vi "Update_PKYK.vi"(8 "error in (no error)":errorcluster, 10 "PokaYoke In":T1 {"MachineCode" items=["MCIG", "MCPC", "MCSA", "MCCA", "MCAC", "MCLA", "MCCM", "MCSC", "MCPA", "MCLP", "MCHP", "MCBC", "MCFA", "MCSR", "MCFV"]; "ExpiryDate" format="%<%I:%M:%S%3u %p\n%d-%m-%Y>T"; "EntDt" format="%<%I:%M:%S%3u %p\n%d-%m-%Y>T"; "UpdDt" format="%<%I:%M:%S%3u %p\n%d-%m-%Y>T"}, 11 "Refnum in":T6) -> (0 "error out":errorcluster, 2 "PokaYoke Out":T1 {"MachineCode" items=["MCIG", "MCPC", "MCSA", "MCCA", "MCAC", "MCLA", "MCCM", "MCSC", "MCPA", "MCLP", "MCHP", "MCBC", "MCFA", "MCSR", "MCFV"]; "ExpiryDate" format="%<%I:%M:%S%3u %p\n%d-%m-%Y>T"; "EntDt" format="%<%I:%M:%S%3u %p\n%d-%m-%Y>T"; "UpdDt" format="%<%I:%M:%S%3u %p\n%d-%m-%Y>T"}, 3 "Refnum out":T6)   [LabVIEW 2020]
uses:
  <vilib>/addons/database/Connection.llb/Conn ObjectReference.ctl
  Controls/Line_PKYK.ctl
  Controls/PARA_CONTROL_STR.ctl
  Controls/PKYK_MCODE.ctl
  Controls/PKYK_DATE.ctl
  Controls/PKYK_Result.ctl
  <userlib>/_OpenG.lib/array/array.llb/Delete Elements from 1D Array (String)__ogtk.vi
  <vilib>/addons/database/NI_Database_API.lvlib
panel:
  out "Format String Name":string[](array[string])
  out "resulting string":string
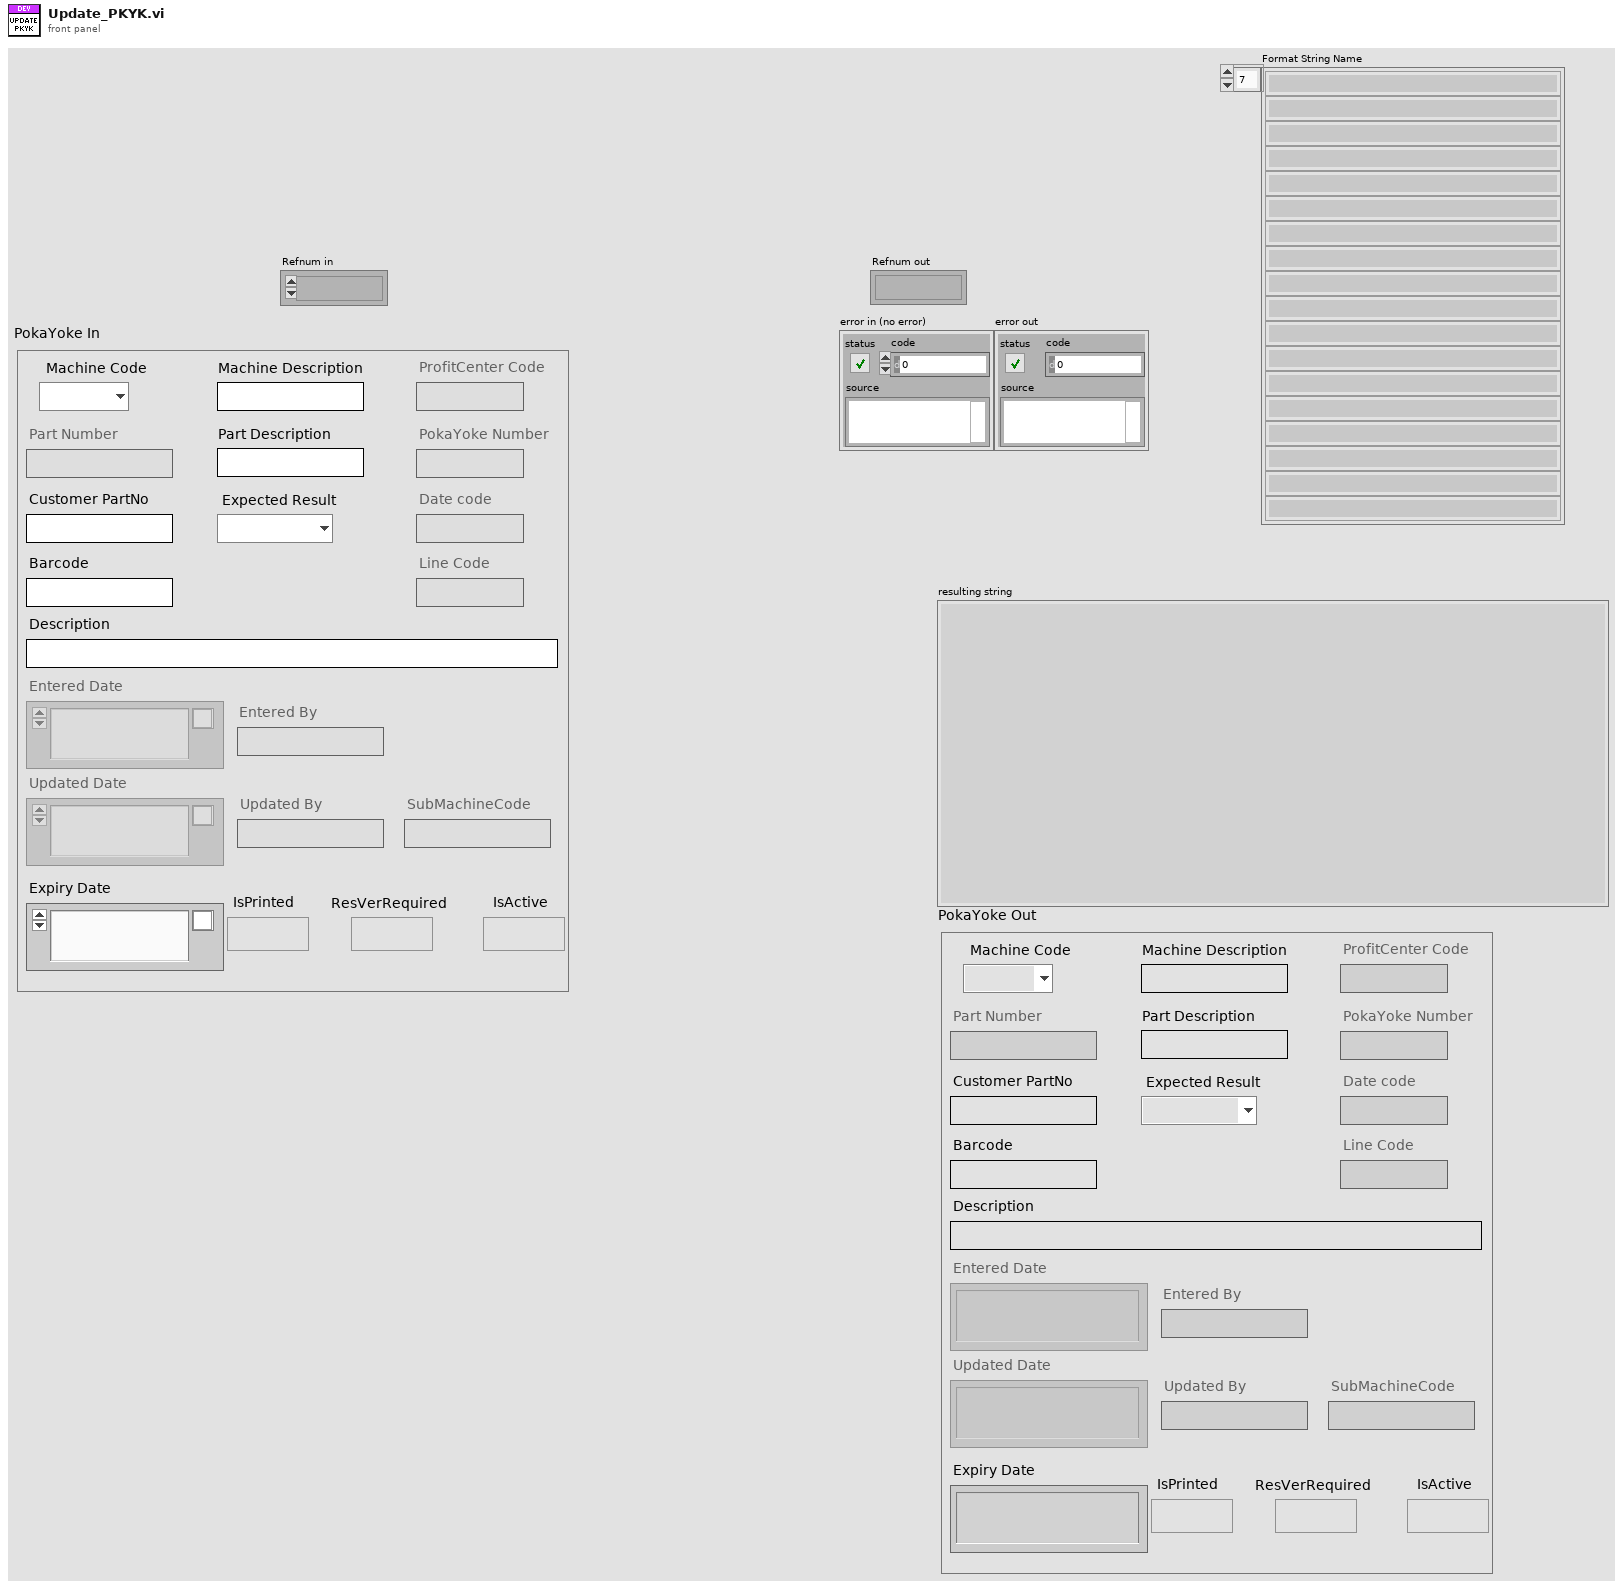
[diagram p1: front panel]
types:
  T1 = typedef "Line_PKYK.ctl" = cluster{"ProfitCenterCode":string, "LineCode":string, "Datecode":string, "PartNumber":T2, "PartDescription":T2, "CustPartNo":T2, "MachineCode":T3, "MachineDescription":T2, "PokaYokeNumber":string, "Description":string, "ExpiryDate":T4, "Barcode":T2, "IsPrinted":bool, "IsActive":bool, "EntBy":T2, "EntDt":T4, "UpdBy":T2, "UpdDt":T4, "ExpResult":T5, "ResVerRequired":bool, "SubMachineCode":T2}
  T2 = typedef "PARA_CONTROL_STR.ctl" = string
  T3 = typedef "PKYK_MCODE.ctl" = u16
  T4 = typedef "PKYK_DATE.ctl" = timestamp
  T5 = typedef "PKYK_Result.ctl" = enum16{"FAIL", "PASS"}
  T6 = typedef "NI_Database_API.lvlib/Conn ObjectReference.ctl" = refnum<k1>
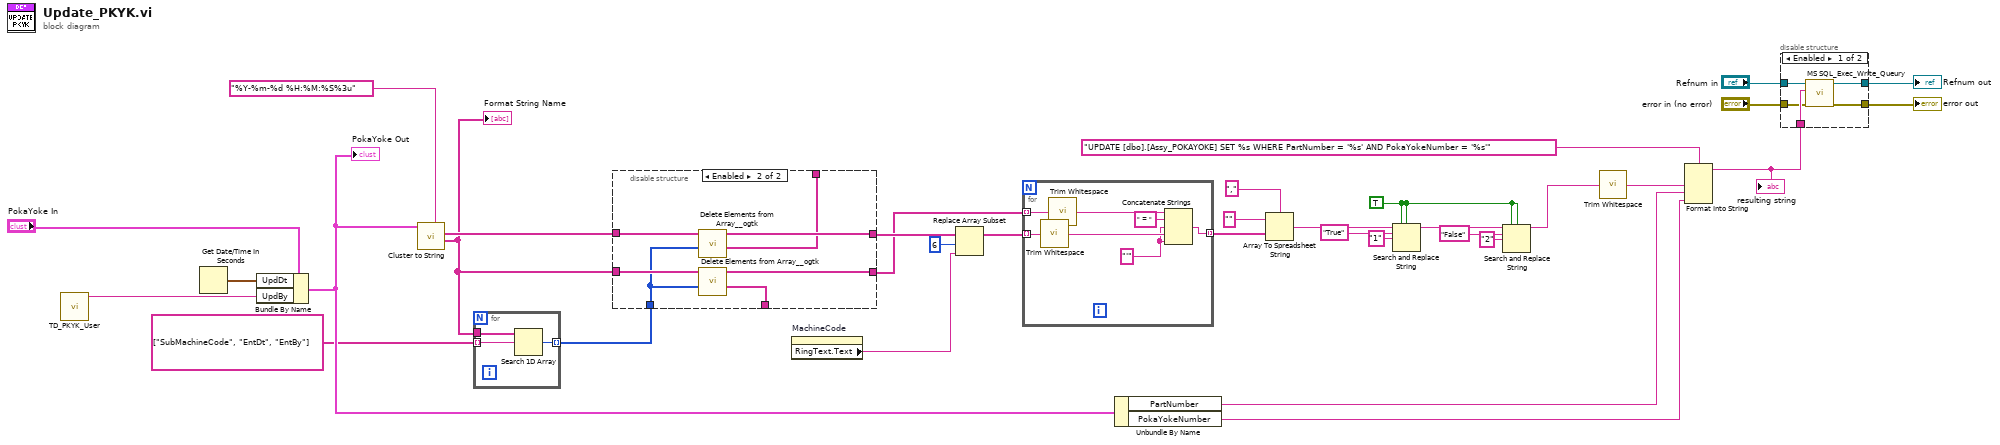
[diagram p0: block diagram]
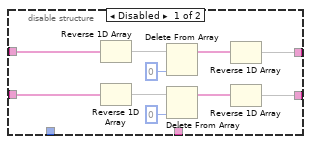
[diagram p2: hidden frame]
diagram:
  w28 = TRUE ("replace all? (F)")
  n1 = call "TD_PKYK_User.vi"() -> ("User"=w1:string)  [unwired: 11 in]
  n2 = Get Date/Time In Seconds() -> (seconds since 1Jan1904=w11:timestamp)
  n3 = Bundle By Name(cluster="PokaYoke In", "UpdDt"=w11, "UpdBy"=w1) -> (w7:T1)
  "PokaYoke Out" <- w7
  n4 = call <userlib>:"Cluster to String.vi"("Time Format String"="%Y-%m-%d %H:%M:%S%3u" ("time format string (%c)"), "Variant In"=w7) -> ("Format String Name"=w4:string[], "Format String Array"=w13:string[])  [unwired: 6 in, 2 out]
  "Format String Name" <- w4
  n5 = for {
    tunnel: w4 -> [w37]
    tunnel: string[] ["SubMachineCode", "EntDt", "EntBy"] ("Format String Name 2") -> [w36] mode=indexing
    tunnel: [w35] -> w2 mode=indexing
    n6 = Search 1D Array(1D array=w37, element=w36) -> (index of element=w35:i32)  [unwired: 1 in]
  }
  n7 = disable-structure shown="Enabled" {
    disable-tunnel: w13 -> [w47 w54]
    disable-tunnel: [w43 w53] -> w12
    disable-tunnel: w4 -> [w39 w51]
    disable-tunnel: [w38 w49] -> w8
    disable-tunnel: w2 -> [_ w50]
    disable-tunnel: [_ w52] -> _
    disable-tunnel: [_ w48] -> _
    frame Disabled {
      n8 = Reverse 1D Array(array=w47) -> (reversed array=w46:string[])
      n9 = Reverse 1D Array(array=w39) -> (reversed array=w40:string[])
      n10 = Delete From Array(array=w46, index=0) -> (array with subset deleted=w44:string[])  [unwired: 1 in, 1 out]
      n11 = Delete From Array(array=w40, index=0) -> (array with subset deleted=w42:string[])  [unwired: 1 in, 1 out]
      n12 = Reverse 1D Array(array=w44) -> (reversed array=w43:string[])
      n13 = Reverse 1D Array(array=w42) -> (reversed array=w38:string[])
    }
    frame Enabled {
      n14 = call-poly <userlib>:"Delete Elements from Array__ogtk.vi"("indices"=w50, "array"=w54) -> ("deleted elements"=w52:string[], "array w/ subset deleted"=w53:string[])  [unwired: 8 in]
      n15 = call-poly <userlib>:"Delete Elements from Array__ogtk.vi"("indices"=w50, "array"=w51) -> ("deleted elements"=w48:string[], "array w/ subset deleted"=w49:string[])  [unwired: 8 in]
    }
  }
  n16 = property on="MachineCode" class="Ring (strict)"() -> ("RingText.Text"=w16:string)  [unwired: 2 in, 2 out]
  n17 = Replace Array Subset(array=w12, new element=w16, index=6) -> (w14:string[])
  n18 = for {
    tunnel: w14 -> [w61] mode=indexing
    tunnel: [w58] -> w15 mode=indexing
    tunnel: w8 -> [w57] mode=indexing
    w59 = "'" ("string")
    n19 = call <vilib>:"Trim Whitespace.vi"("string"=w61) -> ("trimmed string"=w60:string)  [unwired: 1 in]
    n20 = call <vilib>:"Trim Whitespace.vi"("string"=w57) -> ("trimmed string"=w56:string)  [unwired: 1 in]
    n21 = Concatenate Strings(w56, " = " ("string"), w59, w60, w59) -> (w58:string)
  }
  n22 = Unbundle By Name(w7) -> ("PartNumber"=w6:T2, "PokaYokeNumber"=w5:string)
  n23 = Array To Spreadsheet String(delimiter (Tab)=",", array=w15, 3:"" ("format string")) -> (spreadsheet string=w25:string)
  n24 = Search and Replace String(replace all?=w28, case sensitive?=w28, input string=w25, search string="True", replace string="1" ("replace string (\"\")")) -> (result string=w29:string)  [unwired: 3 in, 3 out]
  n25 = Search and Replace String(replace all?=w28, case sensitive?=w28, input string=w29, search string="False", replace string="2" ("replace string (\"\")")) -> (result string=w23:string)  [unwired: 3 in, 3 out]
  n26 = call <vilib>:"Trim Whitespace.vi"("string"=w23) -> ("trimmed string"=w9:string)  [unwired: 1 in]
  n27 = Format Into String(format string="UPDATE [dbo].[Assy_POKAYOKE] SET %s WHERE PartNumber = '%s' AND PokaYokeNumber = '%s'", w9, w6, w5) -> (resulting string=w22:string)  [unwired: 2 in, 1 out]
  "resulting string" <- w22
  n28 = disable-structure shown="Enabled" {
    disable-tunnel: w22 -> [w66 _]
    disable-tunnel: "Refnum in" -> [w65 w67]
    disable-tunnel: [w64 w67] -> w20
    disable-tunnel: "error in (no error)" -> [w63 _]
    disable-tunnel: [w62 _] -> w18
    frame Enabled {
      n29 = call "MS SQL_Exec_Write_Queury.vi"("error in (no error)"=w63, "Query"=w66, "Refnum in"=w65) -> ("error out"=w62:errorcluster, "Refnum out"=w64:T6)  [unwired: 7 in]
    }
    frame Disabled {
    }
  }
  "Refnum out" <- w20
  "error out" <- w18
